vi "CH_LM Flush with Lock.vi"(0 "Meter Index":i32, 5 "error in (no error)":errorcluster, 7 "Lock Timeout / ms (1000)":i32=1000) -> (13 "Lock timed out":bool, 14 "Meter Index":i32, 19 "error out":errorcluster)   [LabVIEW 2017, in "CH_LM.lvlib"]
doc: "This VI is used to flush the read buffer after stopping the streaming mode."
uses:
  CH_LM.lvlib
  CH_LM Action Enumeration.ctl
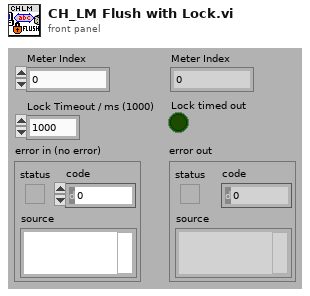
[diagram p1: front panel]
types:
  T1 = typedef "CH_LM.lvlib/CH_LM Action Enumeration.ctl" = enum16{"add", "read", "read by serial", "set", "remove", "delete", "Clear Shift-Register", ""}
  T2 = typedef "CH_LM.lvlib/CH_LM Communication Mode.ctl" = enum16{"None", "USB", "GPIB", "RS232"}
  T3 = typedef "Semaphore RefNum" = refnum<k1>
  T4 = typedef "CH_LM.lvlib/CH_LM Meter Info.ctl" = cluster{"Meter Index":i32, "Serial Number":string, "Queue Cluster":T5, "Data Header":bool, "Data Tokens":T6[]}
  T5 = typedef "CH_LM.lvlib/CH_LM Queue Cluster.ctl" = cluster{"Streaming Queue":refnum<queue>, "Asynch Notifier":refnum<notifier>}
  T6 = typedef "CH_LM.lvlib/CH_LM Data Token.ctl" = enum16{"Raw data", "Quad distance", "Formated data", "Unit", "Pulse period", "Flags", "Sequence ID"}
  T7 = typedef "CH_LM.lvlib/CH_LM Streaming Data.ctl" = cluster{"Value":sgl, "Quad Distance":cluster{"X":sgl, "Y":sgl}, "Display Data":cluster{"Format ID":u8, "Scale ID":u8}, "Unit ID":u8, "Flags":u32, "Pulse Period":u32, "Sequence ID":u32, "Unit String":string}
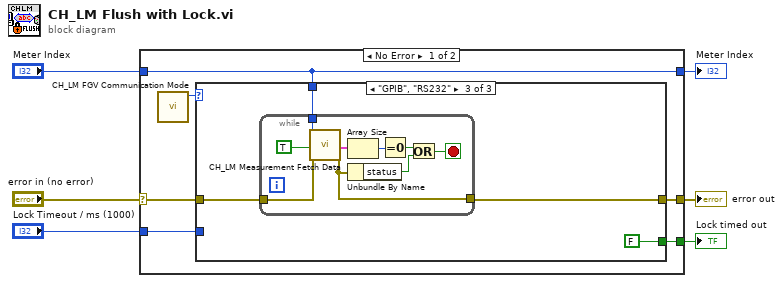
[diagram p0: block diagram]
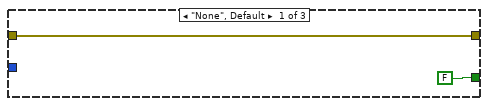
[diagram p2: hidden frame]
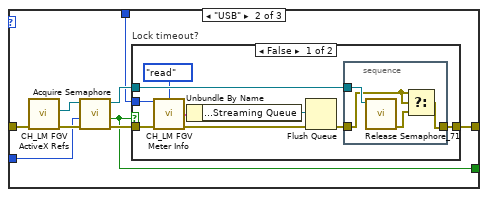
[diagram p3: hidden frame]
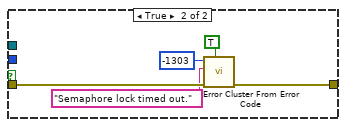
[diagram p4: hidden frame]
diagram:
  n1 = case shown="No Error" "error in (no error)" {
    selector: "error in (no error)" -> [w11 w56]
    tunnel: [w12 w56] -> w6
    tunnel: "Meter Index" -> [w10 w55]
    tunnel: [w10 w55] -> w3
    tunnel: "Lock Timeout / ms (1000)" -> [w9 _]
    tunnel: [w8 _] -> w1
    frame No Error {
      n2 = call "CH_LM FGV Communication Mode.vi"() -> ("Communication Mode"=w7:T2)  [unwired: 3 in, 5 out]
      n3 = case shown="\"GPIB\", \"RS232\"" w7 {
        tunnel: [w14 w23 w42] -> w12
        tunnel: w11 -> [w14 w21 w44]
        tunnel: w10 -> [_ w17 w45]
        tunnel: w9 -> [_ w16 _]
        tunnel: [FALSE ("timed out") w15 FALSE ("timed out")] -> w8
        frame "None", Default {
        }
        frame "USB" {
          n4 = call "CH_LM FGV ActiveX Refs.vi"("error in (no error)"=w21) -> ("error out"=w20:errorcluster, "CH_LM semaphore"=w19:T3)  [unwired: 4 in, 2 out]
          n5 = call <vilib>:"Acquire Semaphore.vi"("error in (no error)"=w20, "ms timeout (-1)"=w16, "semaphore"=w19) -> ("error out"=w22:errorcluster, "timed out"=w15:bool, "semaphore out"=w18:T3)  [unwired: 2 out]
          n6 = case "Lock timeout?" shown="False" w15 {
            tunnel: [w32 w40] -> w23
            tunnel: w17 -> [w31 _]
            tunnel: w22 -> [w30 w39]
            tunnel: w18 -> [w29 _]
            frame False {
              n7 = call "CH_LM FGV Meter Info.vi"("Meter Index"=w31, "Action (read)"=CH_LM_Action_Enumeration."read", "error in (no error)"=w30) -> ("Meter Info"=w27:T4, "error out"=w25:errorcluster)  [unwired: 2 in, 9 out]
              n8 = Unbundle By Name(w27) -> ("Queue Cluster.Streaming Queue"=w26:refnum<queue>)
              n9 = Flush Queue(queue=w26, error in (no error)=w25) -> (error out=w28:errorcluster)  [unwired: 2 out]
              n10 = stacked-sequence {
                tunnel: [w35] -> w32
                tunnel: w29 -> [w34]
                tunnel: w28 -> [w33]
                frame #0 {
                  n11 = call <vilib>:"Release Semaphore_71.vi"("semaphore"=w34) -> ("error out"=w36:errorcluster)  [unwired: 1 in, 5 out]
                  n12 = Select(t=w33, s=w33, f=w36) -> (s? t:f=w35:errorcluster)
                }
              }
            }
            frame True {
              n13 = call <vilib>:"Error Cluster From Error Code.vi"("show call chain? (False)"=TRUE, "error in (no error)"=w39, "error message (\"\")"="Semaphore lock timed out." ("error message (\"\")"), "error code (0)"=-1303) -> ("error out"=w40:errorcluster)  [unwired: 5 out]
            }
          }
        }
        frame "GPIB", "RS232" {
          n14 = while {
            tunnel: w45 -> [w54]
            tunnel: w44 -> [w52]
            tunnel: [w48] -> w42
            stop <- w46 stop-if-true
            n15 = call "CH_LM Measurement Fetch Data.vi"("Meter Index"=w54, "All Records? (F)"=TRUE, "error in (no error)"=w52) -> ("Data Array"=w51:T7[], "error out"=w48:errorcluster)  [unwired: 15 out]
            n16 = Array Size(array=w51) -> (size(s)=w50:i32)
            n17 = Unbundle By Name(w48) -> ("status"=w47:bool)
            n18 = Equal To 0?(x=w50) -> (x = 0?=w49:bool)
            n19 = Or(x=w49, y=w47) -> (x .or. y?=w46:bool)
          }
        }
      }
    }
    frame Error {
    }
  }
  "error out" <- w6
  "Meter Index" <- w3
  "Lock timed out" <- w1
